vi "Core Write DAQ FIFO.vi"(6 "FIFO Timestamps":T2, 8 "error in (no error)":errorcluster, 9 "Timeout (ms)":i32=100, 10 "DAQ In":T1[](array[typedef]), 11 "CIFTag in":refnum<class "CIF_NIChn_Fifo_DAQ.lvclass">) -> (0 "error out":errorcluster, 1 "timed out?":bool, 2 "DAQ Out":T1[](array[typedef]), 3 "CIFTag out":refnum<class "CIF_NIChn_Fifo_DAQ.lvclass">)   [LabVIEW 2021, in "CIF_NIChn_Fifo_DAQ.lvclass"]
uses:
  CIF_NIChn_Fifo_DAQ.lvclass
  D:/dev/CIF-LVCore/src/Channels/CIF_NIChn/NIChn/CIF_NIChn.lvclass
  ChannelCommon/typedef/TimeStamps.ctl
  ChannelCommon/typedef/Datatype Waveform.ctl
  CIF_NIChn_Fifo_DAQ.lvclass/CIF_NIChn_Fifo_DAQ.ctl
  ChannelCommon/CIFFIFO/CIFfifo.lvclass/CIFfifo.ctl
  NIChn/CIF_NIChn.lvclass/CIF_NIChn.ctl
  <vilib>/CIFChannels/Top Level/Write Variable Length U8 Array.vi
  NIChn/Accessors/Read CIF Channel.vi
  NIChn/Accessors/Write CIF Channel.vi
  Flatten.vi
  ChannelCommon/CIFFIFO/Accessors/Read Length.vi
  <vilib>/CIFChannels/SubVIs/Get dll Path.vi
  ChannelCommon/CIFFIFO/Utilities/Update Header.vi
  ChannelCommon/CIFFIFO/Flatten/DVR Flatten.vi
  ChannelCommon/CIFFIFO/Accessors/Write T0.vi
  ChannelCommon/CIFFIFO/Accessors/Write T_Out.vi
  ChannelCommon/CIFFIFO/Accessors/Write ClockID.vi
  <vilib>/CIF Foundation/CIF Utilities/Time/System Time/Get System Time.vi
  ChannelCommon/Utilities/Flatten Header.vi
  ChannelCommon/CIFFIFO/Flatten/DVR Flatten.vi/6fdbece9-bad6-4a8e-9bf7-fe1528478dd6.vi
  ChannelCommon/CIFFIFO/Accessors/Write Payload Length.vi
  ChannelCommon/CIFFIFO/Accessors/Read Header.vi
  <vilib>/CIF Foundation/CIF Utilities/Time/System Time/LabVIEW Time to TAI Time.vi
  CIFCore/Common/Utilities/Add Error.vi
  ChannelCommon/CIFFIFO/Flatten/DVR Flatten.vi/6fdbece9-bad6-4a8e-9bf7-fe1528478dd6.vi/c28b0ead-42ad-4072-80a2-aca7f2bd7ce3.vi
  <vilib>/CIF Foundation/CIF Utilities/Errors/Append Error Location.vi
  ChannelCommon/ChannelCommon.lvlib
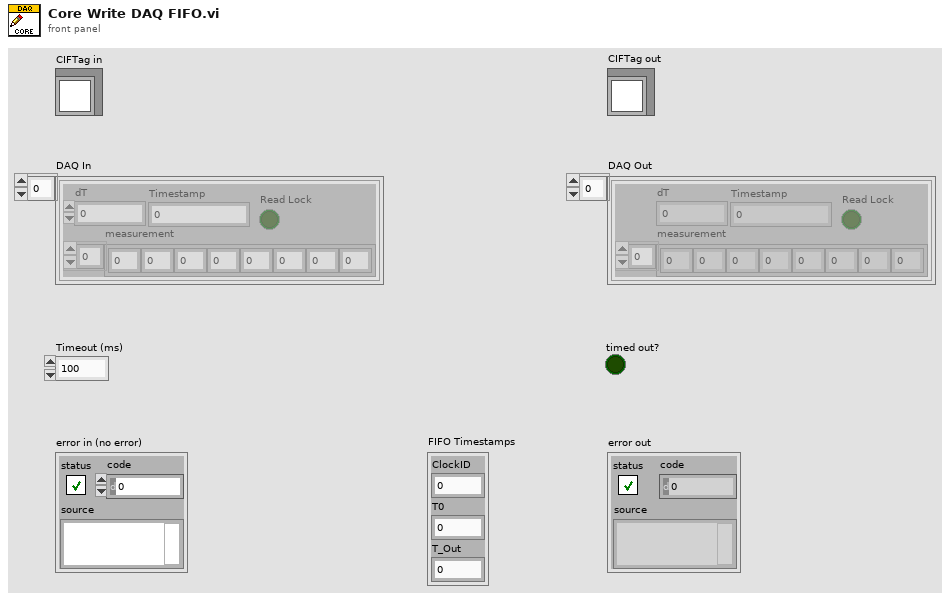
[diagram p1: front panel]
types:
  T1 = typedef "ChannelCommon.lvlib/Datatype Waveform.ctl" = cluster{"measurement":dbl[], "dT":dbl, "Timestamp":u64, "Read Lock":bool}
  T2 = typedef "ChannelCommon.lvlib/TimeStamps.ctl" = cluster{"ClockID":u8, "T0":i64, "T_Out":i64}
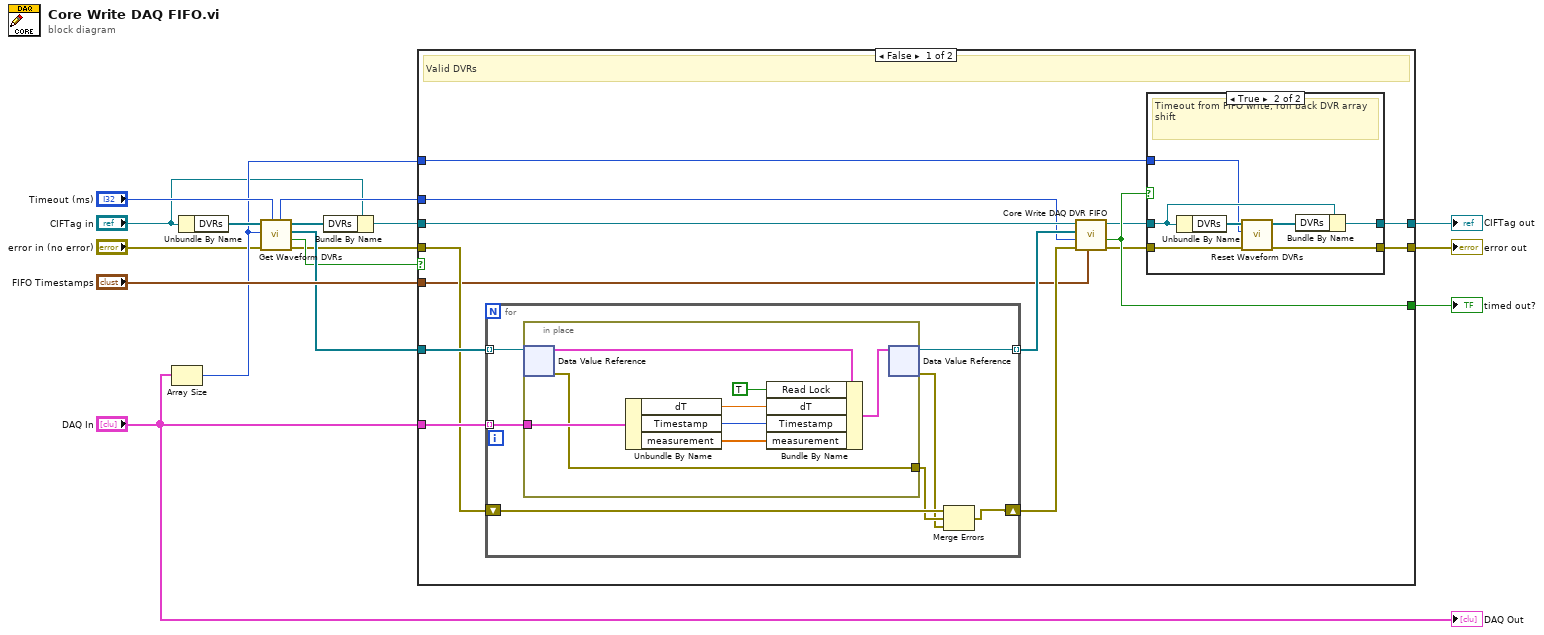
[diagram p0: block diagram]
diagram:
  n1 = Array Size(array="DAQ In") -> (size(s)=w3:i32)
  n2 = Unbundle By Name("CIFTag in") -> ("DVRs"=w12:refnum<data-value>[])
  n3 = call "Get Waveform DVRs.vi"("Timeout in (ms)"="Timeout (ms)", "error in (no error)"="error in (no error)", "Number of Waveforms"=w3, "DVR Circular Buffer in"=w12) -> ("error out"=w6:errorcluster, "Timeout"=w7:bool, "DVRs"=w8:refnum<data-value>[], "DVR Circular Buffer out"=w11:refnum<data-value>[], "Remaining timeout (ms)"=w5:i32)  [unwired: 3 in]
  n4 = Bundle By Name(cluster="CIFTag in", "DVRs"=w11) -> (w9:refnum<class "CIF_NIChn_Fifo_DAQ.lvclass">)
  n5 = case shown="False" w7 {
    selector: w7 -> [_ w55]
    tunnel: w6 -> [w27 w56]
    tunnel: w9 -> [w30 w57]
    tunnel: w8 -> [w29 _]
    tunnel: [w20 w57] -> w16
    tunnel: [w22 w55] -> w15
    tunnel: [w18 w56] -> w14
    tunnel: "DAQ In" -> [w28 _]
    tunnel: "FIFO Timestamps" -> [w24 _]
    tunnel: w5 -> [w23 _]
    tunnel: w3 -> [w17 _]
    frame False {
      # "Valid DVRs"
      n6 = for {
        tunnel: w29 -> [w46] mode=indexing
        tunnel: w28 -> [w45] mode=indexing
        tunnel: [w44] -> w25 mode=indexing
        shift-right: [w40] -> w26
        shift-left: w27 -> [w43]
        n7 = in-place {
          in-place-border: w45 -> [w51]
          in-place-border: [w49] -> w42
          n8 = in-place-dvr #1(w46) -> (w54:T1, w49:errorcluster)
          n9 = Unbundle By Name(w51) -> ("dT"=w53:dbl, "Timestamp"=w52:u64, "measurement"=w47:dbl[])
          n10 = Bundle By Name(cluster=w54, "Read Lock"=TRUE, "dT"=w53, "Timestamp"=w52, "measurement"=w47) -> (w50:T1)
          n11 = in-place-dvr #1(w50) -> (w44:refnum<data-value>, w41:errorcluster)
        }
        n12 = Merge Errors(w43, w42, w41) -> (w40:errorcluster)
      }
      n13 = call "Core Write DAQ DVR FIFO.vi"("FIFO Timestamps"=w24, "error in (no error)"=w26, "Timeout (ms)"=w23, "Data In"=w25, "CIFTag in"=w30) -> ("error out"=w19:errorcluster, "timed out?"=w22:bool, "CIFTag out"=w21:refnum<class "CIF_NIChn_Fifo_DAQ.lvclass">)  [unwired: 3 in, 1 out]
      n14 = case shown="True" w22 {
        tunnel: w21 -> [w32 w39]
        tunnel: [w32 w38] -> w20
        tunnel: w19 -> [w31 w37]
        tunnel: [w31 w36] -> w18
        tunnel: w17 -> [_ w33]
        frame False {
        }
        frame True {
          # "Timeout from FIFO write, roll back DVR array shift"
          n15 = Unbundle By Name(w39) -> ("DVRs"=w34:refnum<data-value>[])
          n16 = call "Reset Waveform DVRs.vi"("error in (no error)"=w37, "Number of Waveforms"=w33, "DVR Circular Buffer in"=w34) -> ("error out"=w36:errorcluster, "DVR Circular Buffer out"=w35:refnum<data-value>[])  [unwired: 7 in]
          n17 = Bundle By Name(cluster=w39, "DVRs"=w35) -> (w38:refnum<class "CIF_NIChn_Fifo_DAQ.lvclass">)
        }
      }
    }
    frame True {
      # "Timeout getting unlocked DVRs"
    }
  }
  "error out" <- w14
  "CIFTag out" <- w16
  "timed out?" <- w15
  "DAQ Out" <- "DAQ In"
